vi "Catch1.vi"(8 "Error":errorcluster, 11 "KNR in":T1) -> (0 "error out 4":errorcluster caption="error out", 1 "Circles (Shape Detection 1)":T3(array[cluster]) {"Position"."Y" format="%.2f"; "Position"."X" format="%.2f"}, 2 "Number of Matches (Shape Detection 1)":i32, 3 "KNR out":T1)   [LabVIEW 2013]
uses:
  <userlib>/KNR OS 3.0 LabVIEW Toolkit/Type Definition/KNR3 Reference.ctl
  <userlib>/_FPGA Interface Advanced Tools/FPGA Interface Base/FPGA Interface Base.lvclass
  <userlib>/KNR OS 3.0 LabVIEW Toolkit/Type Definition/Resource.ctl
panel:
  out "配對數":i32
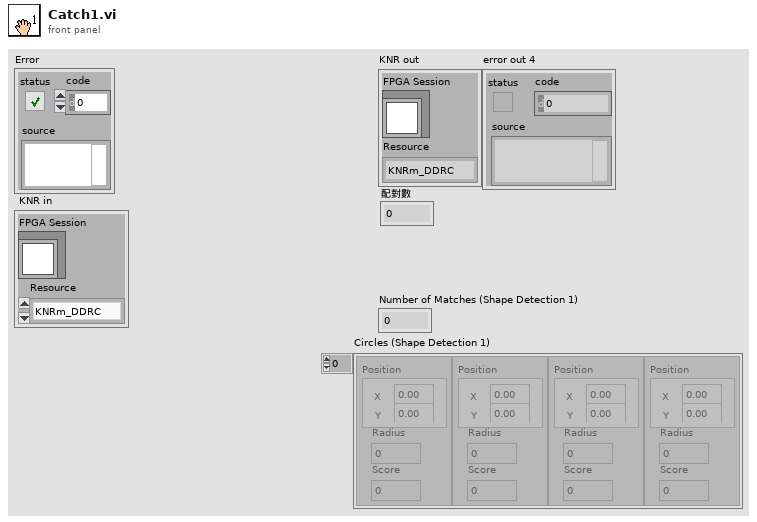
[diagram p1: front panel]
types:
  T1 = typedef "KNR3 Reference.ctl" = cluster{"FPGA Session":refnum<class "FPGA Interface Base.lvclass">, "Resource":T2}
  T2 = typedef "Resource.ctl" = enum16{"KNRm_DDRC", "KNRm_DDDD", "KNRm_DDDR", "KNRm_DDDC", "KNR"}
  T3 = cluster{"Position":cluster{"X":sgl, "Y":sgl}, "Radius":dbl, "Score":dbl}[]
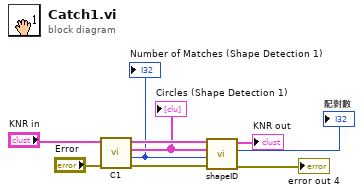
[diagram p0: block diagram]
diagram:
  n1 = call "C1.vi"("Error"="Error", "KNR in"="KNR in") -> ("error out"=w8:errorcluster, "Number of Matches (Shape Detection 1)"=w6:i32, "Circles (Shape Detection 1)"=w7:T3, "KNR out 4"=w9:T1)  [unwired: 5 in, 1 out]
  "Number of Matches (Shape Detection 1)" <- w6
  "Circles (Shape Detection 1)" <- w7
  n2 = call "shapeID.vi"("Error"=w8, "Nb Circles (Circle Detection 1)"=w6, "Circles (Shape Detection 1)"=w7, "KNR in"=w9) -> ("error out 4"=→"error out 4":errorcluster, "配對數"=→"配對數":i32, "KNR out"=→"KNR out":T1)  [unwired: 4 in, 1 out]
